vi "Usage.vi"() -> ()   [LabVIEW 2011, in "Wiimote.lvlib"]
uses:
  Wiimote.lvlib
  Wiimote LEDs.ctl
  Wiimote Acceleration.ctl
panel:
  in  "stop":bool
  out "Nunchuk Acceleration 0G Calibration":T1
  out "Nunchuk Acceleration 1G Calibration":T1
  out "Extension Controller out":bool
  in  "index":i32
  out "Wiimote Acceleration 1G Calibration":T1
  out "Wiimote Acceleration 0G Calibration":T1
  out "Battery Level out":u8
  out "Wiimote LEDs out":T2
  in  "Wiimote LEDs in":T2
  out "error out":errorcluster
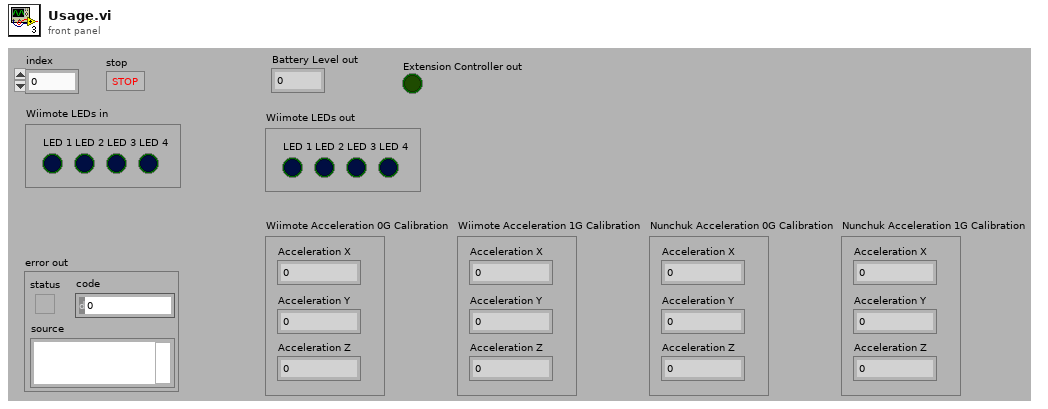
[diagram p1: front panel]
types:
  T1 = typedef "Wiimote.lvlib/Wiimote Acceleration.ctl" = cluster{"Acceleration X":dbl, "Acceleration Y":dbl, "Acceleration Z":dbl}
  T2 = typedef "Wiimote.lvlib/Wiimote LEDs.ctl" = cluster{"LED 1":bool, "LED 2":bool, "LED 3":bool, "LED 4":bool}
  T3 = cluster{"Wiimote 0G Calibration":T1, "Wiimote 1G Calibration":T1, "Nunchuk 0G Calibration":T1, "Nunchuk 1G Calibration":T1}
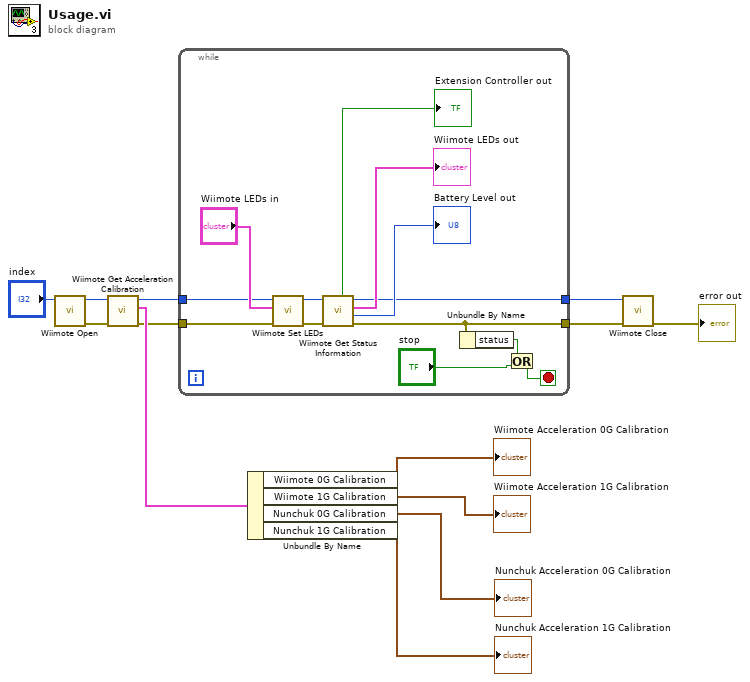
[diagram p0: block diagram]
diagram:
  n1 = call "Wiimote Open.vi"("index"="index") -> ("error out"=w3:errorcluster, "hWiimoteHandle"=w4:u32)  [unwired: 9 in]
  n2 = call "Wiimote Get Acceleration Calibration.vi"("error in"=w3, "hWiimoteHandle in"=w4) -> ("error out"=w1:errorcluster, "Calibration Data Out"=w9:T3, "hWiimoteHandle out"=w2:u32)  [unwired: 7 in]
  n3 = while {
    tunnel: [w24] -> w12
    tunnel: [w17] -> w11
    tunnel: w2 -> [w21]
    tunnel: w1 -> [w20]
    stop <- w16 stop-if-true
    n4 = call "Wiimote Set LEDs.vi"("error in"=w20, "Wiimote LEDs"="Wiimote LEDs in", "hWiimoteHandle in"=w21) -> ("error out"=w19:errorcluster, "hWiimoteHandle out"=w18:u32)  [unwired: 7 in]
    n5 = call "Wiimote Get Status Information.vi"("error in"=w19, "hWiimoteHandle in"=w18) -> ("error out"=w17:errorcluster, "Battery Level out"=→"Battery Level out":u8, "Wiimote LEDs out"=→"Wiimote LEDs out":T2, "hWiimoteHandle out"=w24:u32, "Extension Controller out"=→"Extension Controller out":bool)  [unwired: 5 in]
    n6 = Unbundle By Name(w17) -> ("status"=w15:bool)
    n7 = Or(x=w15, y="stop") -> (x .or. y?=w16:bool)
  }
  n8 = Unbundle By Name(w9) -> ("Wiimote 0G Calibration"=→"Wiimote Acceleration 0G Calibration":T1, "Wiimote 1G Calibration"=→"Wiimote Acceleration 1G Calibration":T1, "Nunchuk 0G Calibration"=→"Nunchuk Acceleration 0G Calibration":T1, "Nunchuk 1G Calibration"=→"Nunchuk Acceleration 1G Calibration":T1)
  n9 = call "Wiimote Close.vi"("error in"=w11, "hWiimoteHandle in"=w12) -> ("error out"=→"error out":errorcluster)  [unwired: 9 in]
